vi "CSGaussmeter.setLower.vi"(0 "i ref in":refnum<vi>, 7 "Lower":dbl, 9 "Unit":T1, 11 "error in (no error)":errorcluster) -> (4 "i ref out":refnum<vi>, 15 "error out":errorcluster)   [LabVIEW 2014, in "CSGaussmeter.lvlib"]
doc: "Dieses VI setzt die Untergrenze für die Limit-Funktion\n\n\nThis VI sets the lower limit for the limit function"
uses:
  CSGaussmeter.lvlib
  instr.lib/FH_55/TypeDef/Unit2.ctl
  CS_Core/CSObj/CSObj.lvlib
  CSlibraries/UtilityLib/UtilityLib.lvlib
  instr.lib/FH_55/FH 55.lvlib
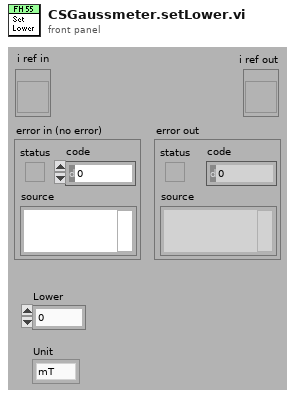
[diagram p1: front panel]
types:
  T1 = typedef "FH 55.lvlib/Unit2.ctl" = enum16{"mT", "G", "kA/m"}
  T2 = typedef "CSGaussmeter.lvlib/CSGaussmeter.i attribute.ctl" = cluster{"Name":string, "VISA Resource Name":refnum<visa-resource-name>, "actValues":cluster{" Limit":bool, "Unit ":T3, "Temp_Unit":T4, "Max":T5, " Filter":bool, " Peak":bool, " Auto_Range":bool, "Range":T6, " Rel":bool, " CTemp":bool, " CField":bool, "AC_DC ":bool, "Set_lower":cluster{"Numeric":dbl, "Cancel Button":bool, "Unit":T1}, "Set_upper":cluster{"Numeric":dbl, "Cancel Button":bool, "Unit":T1}, "Set_Rel":cluster{"Numeric":dbl, "Cancel Button":bool, "Unit":T1}, "Zero":bool, " Local":bool, "Reset":bool, " Init":bool}, "FH 55 Gauss-/Teslameter":T7, "MAX_Value":T8, "MIN_Value":T8, "Rel_Value":T8, "Array ":string[], "LIMU":dbl, " LIML":dbl, "Messwerte 2":string, "Messwerte ":cluster{"Numeric":i32, "OK Button":bool}, "serviceID":cluster{"Current ID":i32, "Unit ID":i32, "Temp ID":i32, "Name ID \n":i32, "Visa ID ":i32}, "setValues ":cluster{" Limit":bool, "Unit ":T3, "Temp_Unit":T4, "Max":T5, " Filter":bool, " Peak":bool, " Auto_Range":bool, "Range":T6, " Rel":bool, " CTemp":bool, " CField":bool, "AC_DC ":bool, "Set_lower":cluster{"Numeric":dbl, "Cancel Button":bool, "Unit":T1}, "Set_upper":cluster{"Numeric":dbl, "Cancel Button":bool, "Unit":T1}, "Set_Rel":cluster{"Numeric":dbl, "Cancel Button":bool, "Unit":T1}, "Zero":bool, " Local":bool, "Reset":bool, " Init":bool}}
  T3 = typedef "FH 55.lvlib/Unit.ctl" = enum16{"T", "G", "A/m"}
  T4 = typedef "FH 55.lvlib/Temp_Unit.ctl" = enum16{"Temp off", "Celsius", "Fahrenheit"}
  T5 = typedef "FH 55.lvlib/Max.ctl" = enum16{"MAX off", "Show MAX", "MAX/MIN"}
  T6 = typedef "FH 55.lvlib/Range.ctl" = enum16{"1", "2", "3", "4", "5", "6", "7"}
  T7 = typedef "FH 55.lvlib/Display.ctl" = cluster{"current value":string, "Limit":string, "Remote":string, "function ":string, "Cluster":cluster{"AC/DC":string, "Auto":string, "Filter":string, "Range":string, "Rel":string, "Peak":string}}
  T8 = typedef "FH 55.lvlib/Value_String.ctl" = cluster{"Numeric":dbl, "String":string}
  T9 = cluster{"Numeric":dbl, "Cancel Button":bool, "Unit":T1}
  T10 = cluster{"VISA Resource Name":refnum<visa-resource-name>}
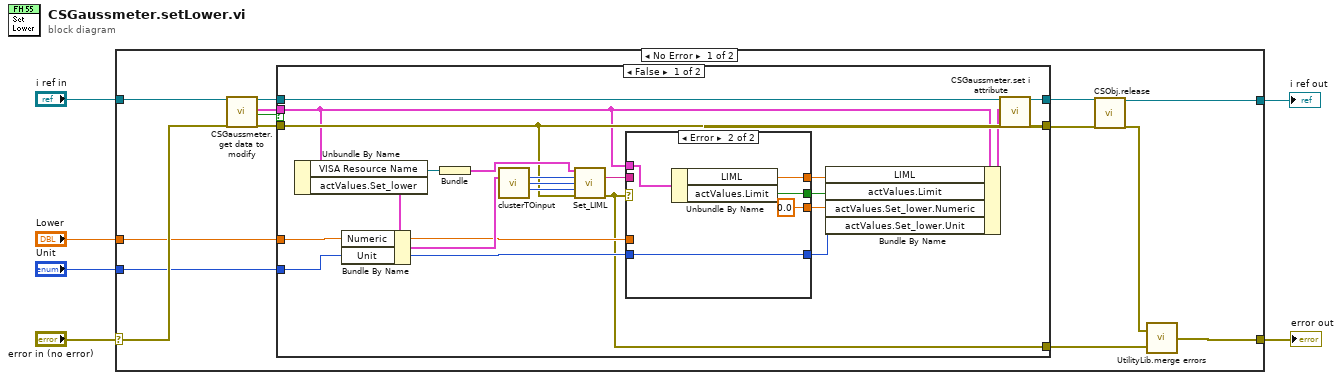
[diagram p0: block diagram]
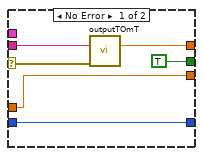
[diagram p2: hidden frame]
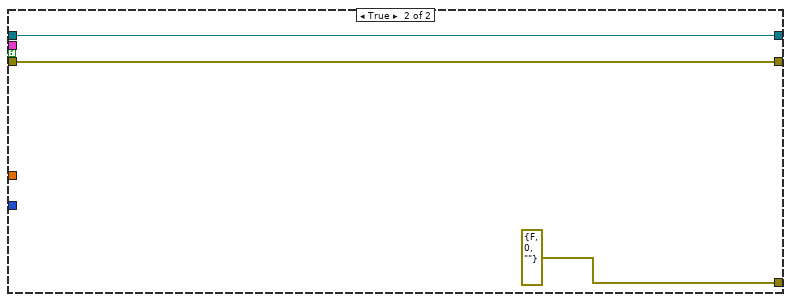
[diagram p3: hidden frame]
diagram:
  n1 = case shown="No Error" "error in (no error)" {
    selector: "error in (no error)" -> [w15 w56]
    tunnel: [w16 w56] -> w3
    tunnel: "i ref in" -> [w14 w57]
    tunnel: [w7 w57] -> w4
    tunnel: "Lower" -> [w8 _]
    tunnel: "Unit" -> [w9 _]
    frame No Error {
      n2 = call "CSGaussmeter.get data to modify.vi"("i ref in"=w14, "error in (no error)"=w15) -> ("i ref out"=w13:refnum<vi>, "i attribute"=w12:T2, "timed out"=w11:bool, "error out"=w10:errorcluster)  [unwired: 14 in]
      n3 = case shown="False" w11 {
        tunnel: w13 -> [w40 w54]
        tunnel: w10 -> [w28 w55]
        tunnel: w12 -> [w21 _]
        tunnel: [w29 w55] -> w18
        tunnel: [w39 w54] -> w20
        tunnel: [w22 errorcluster {"status"=FALSE, "code"=0, "source"=""} ("error out")] -> w17
        tunnel: w9 -> [w24 _]
        tunnel: w8 -> [w25 _]
        frame False {
          n4 = Unbundle By Name(w21) -> ("VISA Resource Name"=w41:refnum<visa-resource-name>, "actValues.Set_lower"=w27:T9)
          n5 = Bundle By Name(cluster=w27, "Numeric"=w25, "Unit"=w24) -> (w33:T9)
          n6 = Bundle("VISA Resource Name"=w41) -> (w34:T10)  [unwired: 1 in]
          n7 = call "clusterTOinput.vi"("Set_Rel"=w33) -> ("Range"=w30:T6, "Numeric"=w31:i32, "Unit"=w32:T3)  [unwired: 11 in, 1 out]
          n8 = call "Set_LIML.vi"("VisaCluster"=w34, "Range"=w30, "Ziffern"=w31, "Unit"=w32, "error in (no error)"=w28) -> ("Answer"=w36:string, "error out"=w22:errorcluster)  [unwired: 8 in, 1 out]
          n9 = case shown="Error" w22 {
            selector: w22 -> [w44 _]
            tunnel: [TRUE ("actValues.Limit") w48] -> w37
            tunnel: w36 -> [w46 _]
            tunnel: [w45 w49] -> w35
            tunnel: [w43 0.0 ("Numeric")] -> w26
            tunnel: w25 -> [w43 _]
            tunnel: w24 -> [w42 w52]
            tunnel: [w42 w52] -> w23
            tunnel: w21 -> [_ w50]
            frame No Error {
              n10 = call "outputTOmT.vi"("Input"=w46, "error in (no error)"=w44) -> ("Numeric"=w45:dbl)  [unwired: 12 in, 1 out]
            }
            frame Error {
              n11 = Unbundle By Name(w50) -> ("LIML"=w49:dbl, "actValues.Limit"=w48:bool)
            }
          }
          n12 = Bundle By Name(cluster=w21, "LIML"=w35, "actValues.Limit"=w37, "actValues.Set_lower.Numeric"=w26, "actValues.Set_lower.Unit"=w23) -> (w38:T2)
          n13 = call "CSGaussmeter.set i attribute.vi"("i ref in"=w40, "i attribute"=w38, "error in (no error)"=w28) -> ("i ref out"=w39:refnum<vi>, "error out"=w29:errorcluster)  [unwired: 15 in]
        }
        frame True {
        }
      }
      n14 = call "CSObj.release.vi"("i ref in"=w20, "error in (no error)"=w18) -> ("i ref out"=w7:refnum<vi>, "error out"=w19:errorcluster)  [unwired: 16 in]
      n15 = call "UtilityLib.merge errors.vi"("error2 (no error)"=w17, "error1 (no error)"=w19) -> ("error out"=w16:errorcluster)
    }
    frame Error {
    }
  }
  "i ref out" <- w4
  "error out" <- w3
